vi "Periodic Tasks.vi"(8 "error in":errorcluster) -> ()   [LabVIEW 2020]
doc: "This VI runs in parallel to other robot code. It can contain as many user-defined periodic loops as you need. These can carry out PID or other sorts of timed response."
uses:
  <vilib>/Analysis/coordinate.llb/Angle Units.ctl
  <vilib>/Analysis/coordinate.llb/Wrap Angle (scalar).vi
  <vilib>/Rock Robotics/WPI/ThirdParty/Phoenix-LabVIEW/Pigeon IMU/CTRE_PigeonIMU_GetYPR.vi
  <vilib>/Rock Robotics/Network Tables/NT Write Number.vi
  <vilib>/Rock Robotics/Network Tables/NT Read Boolean.vi
  <vilib>/Rock Robotics/Network Tables/NT Write Boolean.vi
  Robot Global Data.vi
  <vilib>/Analysis/NI_AAL_Angle.lvlib
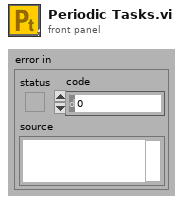
[diagram p1: front panel]
types:
  T1 = typedef "NI_AAL_Angle.lvlib/Angle Units.ctl" = i32
  T2 = typedef "WPI_DriverStationRobotMode2.ctl" = enum16{"Autonomous Disabled", "Autonomous Enabled", "Teleop Disabled", "Teleop Enabled", "Disconnected", "Finish", "Test Disabled", "Test Enabled", "Emergency Stopped"}
  T3 = typedef "WPI_MotorControlDeviceRef.ctl" = cluster{"DeviceStatus":errorcluster, "Type":T4, "PWM":cluster{"PWM Channel":T5, "DeadBand":T6}, "CAN":cluster{"Device Number":u8, "SetOutput VI Ref":variant, "GetOutput VI Ref":variant, "Enable VI Ref":variant, "Disable VI Ref":variant, "Data":variant}, "Invert":bool, "DIO PWM":cluster{"PWM \"Enable\" Channel":T5, "DIOChannel":T7, "PWM Rate":dbl}}
  T4 = typedef "WPI_MotorControlType.ctl" = enum16{"PWM", "CAN", "DIO PWM"}
  T5 = typedef "FPGA_DIOPWMChannel.ctl" = enum8{"PWM 0", "PWM 1", "PWM 2", "PWM 3", "PWM 4", "PWM 5", "PWM 6", "PWM 7", "PWM 8", "PWM 9", "PWM MXP 0", "PWM MXP 1", "PWM MXP 2", "PWM MXP 3", "PWM MXP 4", "PWM MXP 5", "PWM MXP 6", "PWM MXP 7", "PWM MXP 8", "PWM MXP 9", "Invalid"}
  T6 = typedef "WPI_PWMDeadband.ctl" = cluster{"Name":string, "maxPositivePwm":i32, "minPositivePwm":i32, "centerPwm":i32, "maxNegativePwm":i32, "minNegativePwm":i32, "angularRange":u16}
  T7 = typedef "FPGA_DIOChannel.ctl" = enum8{"DIO 0", "DIO 1", "DIO 2", "DIO 3", "DIO 4", "DIO 5", "DIO 6", "DIO 7", "DIO 8", "DIO 9", "DIO MXP 0", "DIO MXP 1", "DIO MXP 2", "DIO MXP 3", "DIO MXP 4", "DIO MXP 5", "DIO MXP 6", "DIO MXP 7", "DIO MXP 8", "DIO MXP 9", "DIO MXP 10", "DIO MXP 11", "DIO MXP 12", "DIO MXP 13", "DIO MXP 14", "DIO MXP 15", "SPI Port CS1", "SPI Port CS2", "SPI Port CS3", "SPI Port MISO", "SPI Port MOSI", "Invalid"}
  T8 = typedef "CTRE_PigeonIMU_DeviceRef.ctl" = cluster{"DeviceStatus":errorcluster, "Device Number":u8, "Type":T9, "Device ID":u32, "Handle":u64, "UsageFrame":u32, "Library Path":path}
  T9 = typedef "CTRE_PigeonIMU_ConnectionType.ctl" = u32
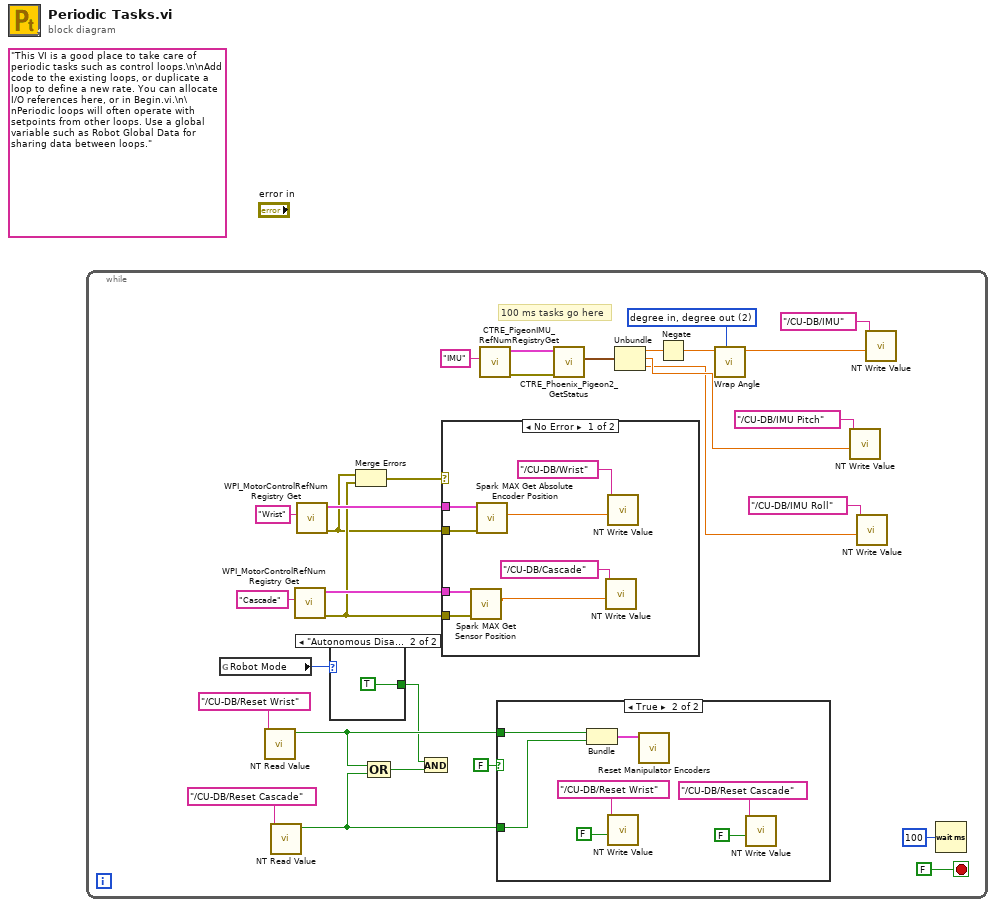
[diagram p0: block diagram]
diagram:
  (unwired) "This VI is a good place to take care of periodic tasks such as control loops.\n\nAdd code to the existing loops, or duplicate a loop to define a new rate. You can allocate I/O references here, or in Begin.vi.\n\nPeriodic loops will often operate with setpoints from other loops. Use a global variable such as Robot Global Data for sharing data between loops."
  n1 = while {
    stop <- FALSE stop-if-true
    w5 = T1 2 items=["radian in, radian out", "radian in, degree out", "degree in, degree out", "degree in, radian out"] ("angle units")
    # "100 ms tasks go here"
    n2 = global read "Robot Global Data.vi" "Robot Mode"() -> (w14:T2)
    n3 = call-poly <vilib>:"NT Read Value.vi"("name"="/CU-DB/Reset Wrist") -> ("value"=w17:bool)  [unwired: 8 in, 2 out]
    n4 = call-poly <vilib>:"NT Read Value.vi"("name"="/CU-DB/Reset Cascade") -> ("value"=w16:bool)  [unwired: 8 in, 2 out]
    n5 = call <vilib>:"WPI_MotorControlRefNum Registry Get.vi"("refnum name"="Cascade") -> ("error out"=w11:errorcluster, "MotorControlDevRef"=w15:T3)  [unwired: 9 in]
    n6 = call <vilib>:"WPI_MotorControlRefNum Registry Get.vi"("refnum name"="Wrist") -> ("error out"=w10:errorcluster, "MotorControlDevRef"=w21:T3)  [unwired: 9 in]
    n7 = case shown="\"Autonomous Disabled\", \"Teleop Disabled\", \"Test Disabled\"" w14 {
      tunnel: [_ TRUE] -> w12
      frame Default {
      }
      frame "Autonomous Disabled", "Teleop Disabled", "Test Disabled" {
      }
    }
    n8 = Merge Errors(w10, w11) -> (w9:errorcluster)
    n9 = Compound Arithmetic op=OR(w17, w16) -> (w13:bool)
    n10 = And(x=w12, y=w13) -> ()  [unwired: 1 out]
    n11 = case shown="No Error" w9 {
      tunnel: w21 -> [w37 _]
      tunnel: w15 -> [w34 _]
      tunnel: w11 -> [w32 _]
      tunnel: w10 -> [w31 _]
      frame No Error {
        n12 = call <vilib>:"Spark MAX Get Sensor Position.vi"("error in (no error)"=w32, "MotorControlDevRef in"=w34) -> ("Sensor Position"=w33:dbl)  [unwired: 6 in, 3 out]
        n13 = call <vilib>:"Spark MAX Get Absolute Encoder Position.vi"("error in (no error)"=w31, "MotorControlDeviceRef in"=w37) -> ("Position"=w36:dbl)  [unwired: 6 in, 3 out]
        n14 = call-poly <vilib>:"NT Write Value.vi"("value"=w33, "name"="/CU-DB/Cascade") -> ()  [unwired: 9 in, 1 out]
        n15 = call-poly <vilib>:"NT Write Value.vi"("value"=w36, "name"="/CU-DB/Wrist") -> ()  [unwired: 9 in, 1 out]
      }
      frame Error {
      }
    }
    n16 = call <vilib>:"CTRE_PigeonIMU_RefNumRegistryGet.vi"("refnum name"="IMU") -> ("error out"=w27:errorcluster, "PigeonIMUDevRef"=w26:T8)  [unwired: 9 in]
    n17 = case shown="True" FALSE {
      tunnel: w17 -> [_ w46]
      tunnel: w16 -> [_ w45]
      frame False {
      }
      frame True {
        n18 = Bundle("value"=w46, "value"=w45) -> (w44:cluster{"value":bool, "value":bool})  [unwired: 1 in]
        n19 = call-poly <vilib>:"NT Write Value.vi"("value"=FALSE, "name"="/CU-DB/Reset Wrist") -> ()  [unwired: 9 in, 1 out]
        n20 = call "Reset Manipulator Encoders.vi"("Reset Parameters"=w44) -> ()  [unwired: 10 in, 1 out]
        n21 = call-poly <vilib>:"NT Write Value.vi"("value"=FALSE, "name"="/CU-DB/Reset Cascade") -> ()  [unwired: 9 in, 1 out]
      }
    }
    n22 = call-poly <vilib>:"CTRE_Phoenix_Pigeon2_GetStatus.vi"("error in (no error)"=w27, "PigeonIMUDevRef"=w26) -> ("Yaw Pitch Roll"=w28:cluster{"Yaw":dbl, "Pitch":dbl, "Roll":dbl})  [unwired: 7 in, 2 out]
    n23 = Unbundle(w28) -> ("Yaw"=w20:dbl, "Pitch"=w2:dbl, "Roll"=w1:dbl)
    n24 = Negate(x=w20) -> (-x=w7:dbl)
    n25 = call-poly <vilib>:"Wrap Angle.vi"("angle units"=w5, "angle in"=w7) -> ("angle out"=w6:dbl)  [unwired: 8 in, 1 out]
    n26 = call-poly <vilib>:"NT Write Value.vi"("value"=w2, "name"="/CU-DB/IMU Pitch") -> ()  [unwired: 9 in, 1 out]
    n27 = call-poly <vilib>:"NT Write Value.vi"("value"=w1, "name"="/CU-DB/IMU Roll") -> ()  [unwired: 9 in, 1 out]
    n28 = call-poly <vilib>:"NT Write Value.vi"("value"=w6, "name"="/CU-DB/IMU") -> ()  [unwired: 9 in, 1 out]
    n29 = Wait (ms)(milliseconds to wait=u32 100) -> ()  [unwired: 1 out]
  }
